vi "Read Grid.vi"(8 "error in (no error)":errorcluster, 11 "GoL in":refnum<class "GoL.lvclass">) -> (0 "error out":errorcluster, 2 "Grid":u8[][](array[numeric]), 3 "GoL out":refnum<class "GoL.lvclass">)   [LabVIEW 2026, in "GoL.lvlib" / "GoL.lvclass"]
uses:
  GoL.lvclass
  GoL.lvclass/GoL.ctl
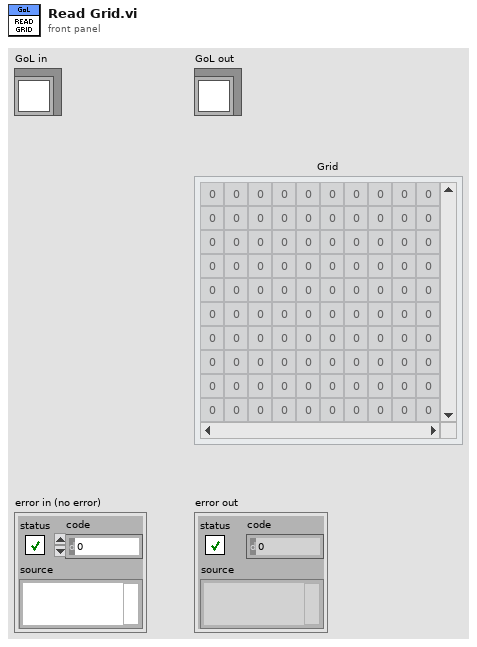
[diagram p1: front panel]
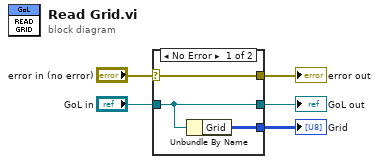
[diagram p0: block diagram]
diagram:
  n1 = case shown="No Error" "error in (no error)" {
    selector: "error in (no error)" -> [w8 w9]
    tunnel: [w8 w9] -> w4
    tunnel: [w7 w10] -> w2
    tunnel: "GoL in" -> [w7 w10]
    tunnel: [w6 _] -> w1
    frame No Error {
      n2 = Unbundle By Name(w7) -> ("Grid"=w6:u8[][])
    }
    frame Error {
    }
  }
  "error out" <- w4
  "GoL out" <- w2
  "Grid" <- w1
